vi "Get Configuration Default.vi"(8 "error in (no error)":errorcluster) -> (0 "error out":errorcluster, 3 "Measurement Configuration Default":T1={"delay"=10.0})   [LabVIEW 2020, in "CancellableMeasurementProxy.lvlib"]
uses:
  CancellableMeasurementProxy.lvlib
  Measurement Configuration.ctl
  e54118e4-a0f5-41b8-bd23-fc2d3fb72aa9.vi
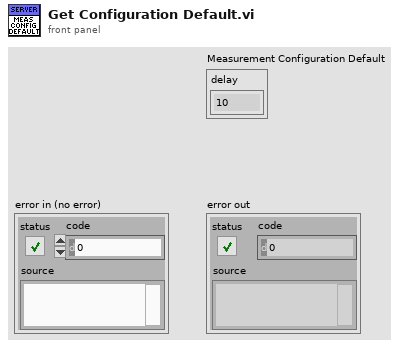
[diagram p1: front panel]
types:
  T1 = typedef "CancellableMeasurementProxy.lvlib/Measurement Configuration.ctl" = cluster{"delay":dbl}
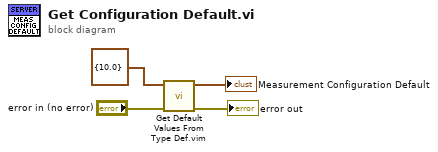
[diagram p0: block diagram]
diagram:
  n1 = call "Get Default Values From Type Def.vim"("error in (no error)"="error in (no error)", "Type Def"=T1 {"delay"=10.0} ("Measurement Configuration")) -> ("error out"=→"error out":errorcluster, "Default Values"=→"Measurement Configuration Default":T1)  [unwired: 8 in]
